vi "thermometersort.vi"() -> ()   [LabVIEW 2022 SP3]
uses:
  002e24af-94bd-407c-8986-31a9b5211204.vi
  <vilib>/Comparison/Less/Less Functor/Less Functor.lvclass
panel:
  in  "stop":bool
  out "Array 2":dbl[](array[numeric])
  in  "Boolean":bool
  out "Array":dbl[](array[numeric])
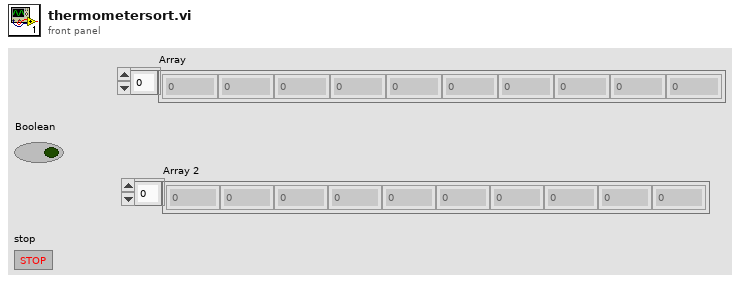
[diagram p1: front panel]
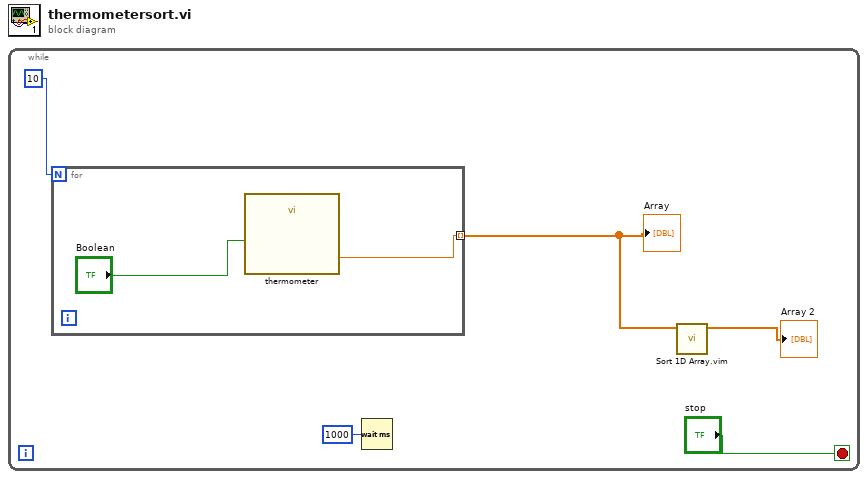
[diagram p0: block diagram]
diagram:
  n1 = while {
    stop <- "stop" stop-if-true
    n2 = for {
      N: 10 -> [_]
      tunnel: [w7] -> w4 mode=indexing
      n3 = call "thermometer.vi"("Temp Scale"="Boolean") -> ("Thermometer"=w7:dbl)
    }
    "Array" <- w4
    n4 = Wait (ms)(milliseconds to wait=u32 1000) -> ()  [unwired: 1 out]
    n5 = call "Sort 1D Array.vim"("unsorted array"=w4) -> ("sorted array"=→"Array 2":dbl[])  [unwired: 10 in]
  }
